vi "PI_GCS3_Configuration_Setup_LimitSwitch.vi"(0 "System no.":i32=1 min=1 step=1, 1 "Conn. Axes":string[](array[string]), 5 "error in":errorcluster) -> (14 "Has\nlimit switch?":bool[](array[boolean]), 19 "error out":errorcluster)   [LabVIEW 2026]
doc: "Check which axes have a limit switch."
uses:
  SpecialCommand/ConfigurationMemoryType.ctl
panel:
  # "Check which axes have a limit switch."
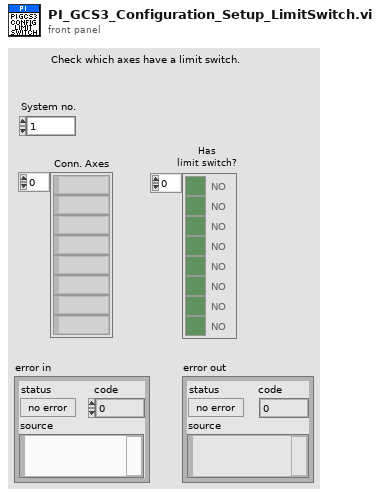
[diagram p1: front panel]
types:
  T1 = typedef "ConfigurationMemoryType.ctl" = enum16{"RAM", "TMP", "FLASH"}
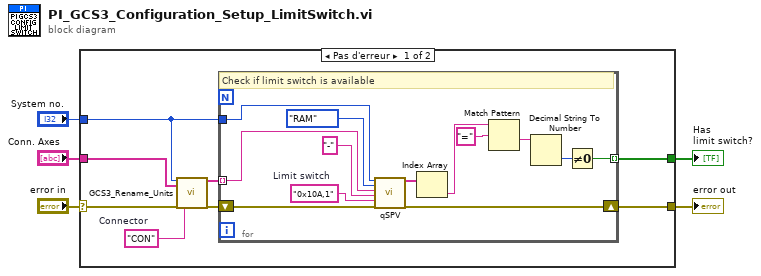
[diagram p0: block diagram]
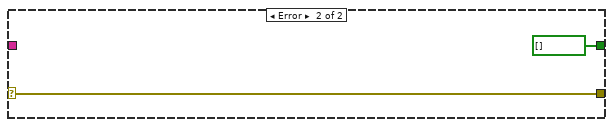
[diagram p2: hidden frame]
diagram:
  n1 = case shown="Pas d'erreur" "error in" {
    selector: "error in" -> [w8 w28]
    tunnel: [w13 w28] -> w2
    tunnel: "Conn. Axes" -> [w9 _]
    tunnel: "System no." -> [w10 _]
    tunnel: [w12 bool[] []] -> w1
    frame No Error {
      w11 = "CON"  # Connector
      n2 = call "GCS3_Rename_Units.vi"("System No."=w10, "Axes"=w9, "error in (no error)"=w8, "Target Unit"=w11) -> ("GCS 3.0 Units"=w6:string[], "error out"=w7:errorcluster)  [unwired: 14 in]
      n3 = for {
        shift-right: [w26] -> w13
        shift-left: w7 -> [w20]
        tunnel: w10 -> [w22]
        tunnel: w6 -> [w24] mode=indexing
        tunnel: [w14] -> w12 mode=indexing
        w25 = "0x10A,1"  # Limit switch
        # "Check if limit switch is available"
        n4 = call "qSPV.vi"("System no."=w22, "Target Memory Type"=ConfigurationMemoryType."RAM", "ContainerUnit"=w24, "FunctionUnit"="-", "ParameterID"=w25, "error in"=w20) -> ("Values"=w18:string[], "error out"=w26:errorcluster)  [unwired: 12 in]
        n5 = Index Array(array=w18) -> (element=w17:string)  [unwired: 1 in]
        n6 = Match Pattern(string=w17, regular expression="=") -> (after substring=w16:string)  [unwired: 1 in, 3 out]
        n7 = Decimal String To Number(string=w16) -> (number=w15:i32)  [unwired: 2 in, 1 out]
        n8 = Not Equal To 0?(x=w15) -> (x != 0?=w14:bool)
      }
    }
    frame Error {
    }
  }
  "error out" <- w2
  "Has\nlimit switch?" <- w1
